vi "Parse POSCAR.vi"(8 "error in (no error)":errorcluster, 10 "POSCAR Type":string(combo)="Unknown", 11 "POSCAR File":path) -> (0 "error out":errorcluster, 1 "Summary Values":string[](array[string])=["# Atoms", "Cell Volume (A^3)", "|C|"], 2 "Summary Headers":string[](array[string])=["# Atoms", "Cell Volume (A^3)", "|A| (Å)", "|B| (Å)", "|C| (Å)", "alpha (deg)", "beta (deg)", "gamma (deg)"], 3 "Structure":T1)   [LabVIEW 2010]
uses:
  <vilib>/Analysis/baseanly.llb/Real Dot Product.vi
  <vilib>/Analysis/_algsub.llb/Real Vector Norm.vi
  <vilib>/Analysis/NI_AALPro.lvlib
  <vilib>/Analysis/NI_AALBase.lvlib
panel:
  out "element":string
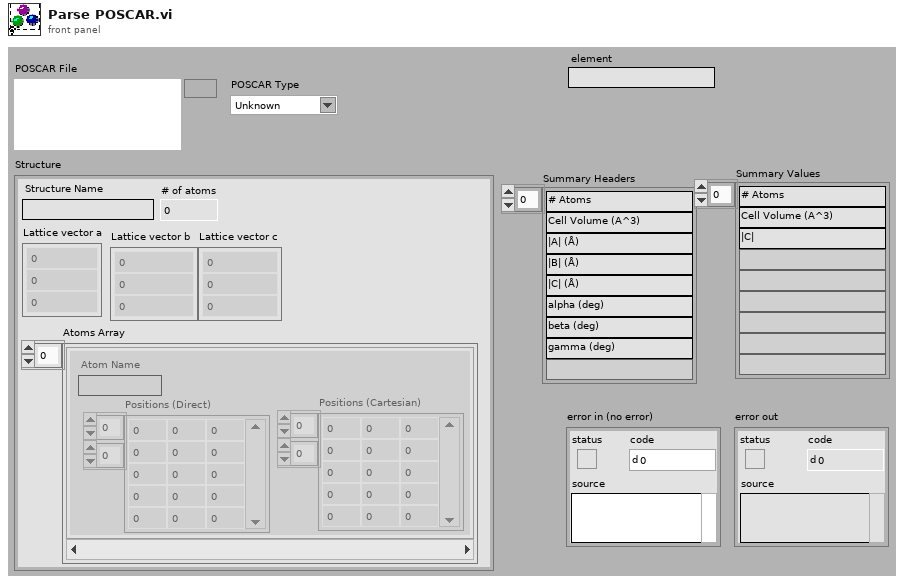
[diagram p1: front panel]
types:
  T1 = cluster{"Structure Name":string, "Lattice vector a":dbl[], "Lattice vector b":dbl[], "Lattice vector c":dbl[], "Atoms Array":cluster{"Atom Name":string, "Positions (Direct)":dbl[][], "Positions (Cartesian)":dbl[][]}[], "# of atoms":i32}
  T2 = cluster{"trimmed string":string, dbl[], dbl[], dbl[], cluster{string, dbl[][], dbl[][]}[], "token string":dbl}
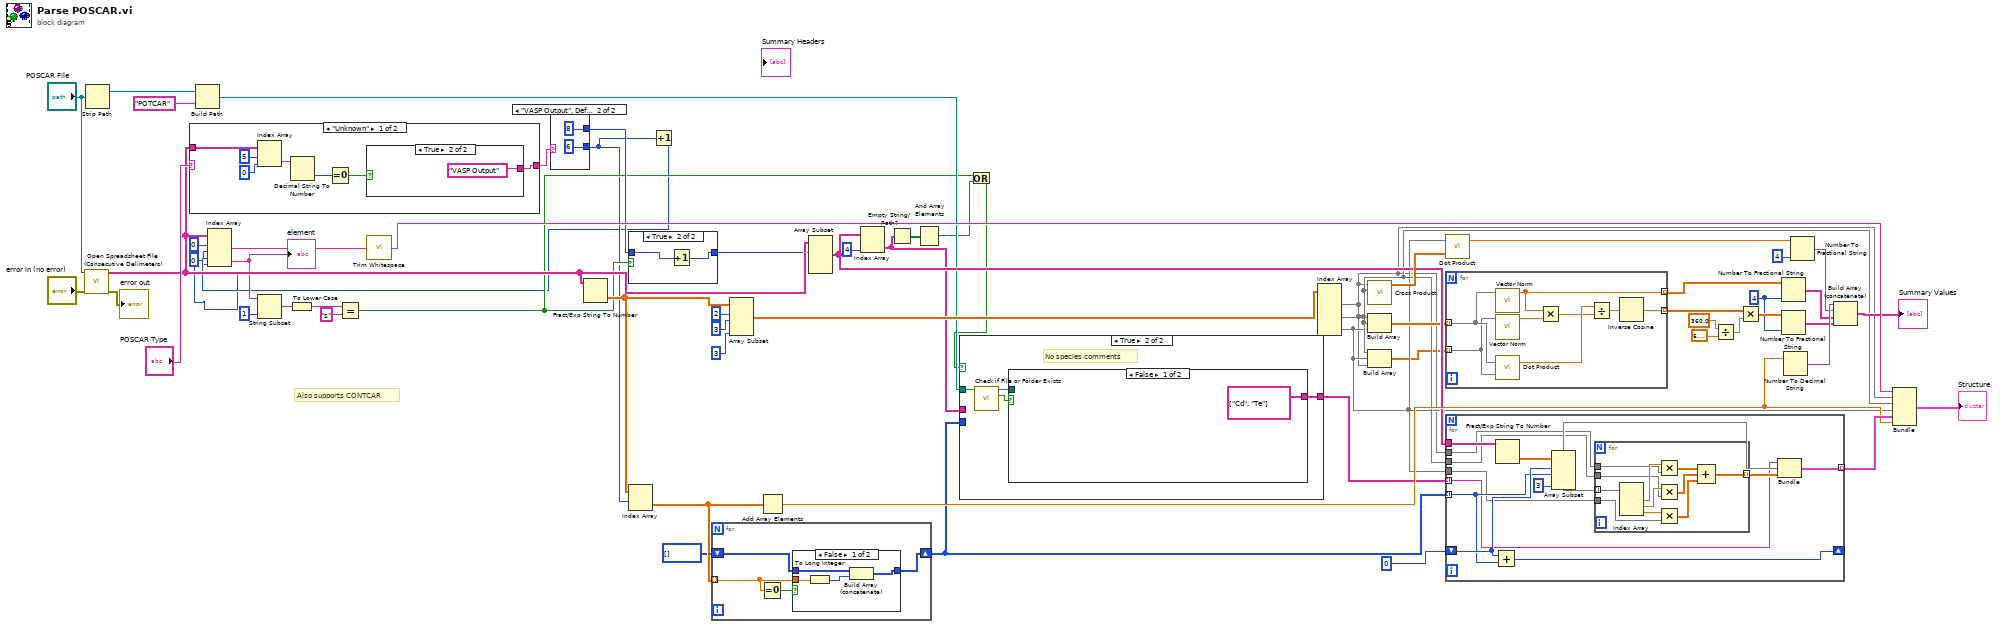
[diagram p0: block diagram]
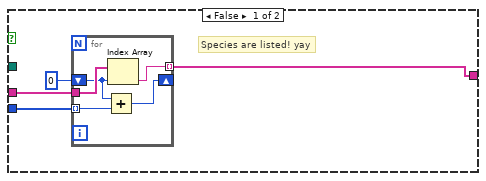
[diagram p3: hidden frame]
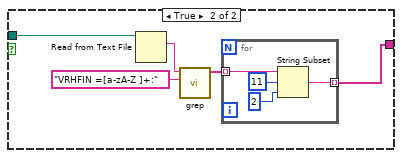
[diagram p4: hidden frame]
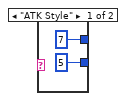
[diagram p6: hidden frame]
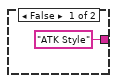
[diagram p7: hidden frame]
diagram:
  w20 = i16 4 ("precision (6)")
  w1 = 0 ("disabled index (col)")
  # "Also supports CONTCAR"
  n1 = call "Open Spreadsheet File (Consecutive Delimeters).vi"("error in (no error)"="error in (no error)", "File"="POSCAR File") -> ("error out"=→"error out":errorcluster, "Array"=w14:string[][])  [unwired: 8 in]
  n2 = Strip Path(path="POSCAR File") -> (stripped path=w40:path)  [unwired: 1 out]
  n3 = case shown="\"Unknown\"" "POSCAR Type" {
    selector: "POSCAR Type" -> [_ w72]
    tunnel: w14 -> [w69 _]
    tunnel: [w63 w72] -> w60
    frame "Unknown" {
      n4 = Index Array(array=w69, index (row)=5, index (col)=0 ("disabled index (col)")) -> (element=w66:string)
      n5 = Decimal String To Number(string=w66) -> (number=w65:i32)  [unwired: 2 in, 1 out]
      n6 = Equal To 0?(x=w65) -> (x = 0?=w64:bool)
      n7 = case shown="True" w64 {
        tunnel: ["ATK Style" "VASP Output"] -> w63
        frame False {
        }
        frame True {
        }
      }
    }
    frame Default {
    }
  }
  n8 = Build Path(base path=w40, name or relative path="POTCAR") -> (appended path=w36:path)
  n9 = case shown="\"VASP Output\", Default" w60 {
    tunnel: [5 ("index (row)") 6 ("index (row)")] -> w3
    tunnel: [7 ("index") 8 ("index")] -> w9
    frame "ATK Style" {
    }
    frame "VASP Output", Default {
    }
  }
  n10 = Fract/Exp String To Number(string=w14) -> (number=w15:dbl[][])  [unwired: 3 in, 1 out]
  n11 = Index Array(array=w15, index (row)=w3) -> (element=w59:dbl[])  [unwired: 1 in]
  n12 = Increment(x=w3) -> (x+1=w2:i32)
  n13 = Index Array(array=w14, index (row) #1=0 ("index (row)"), index (col) #1=w1, index (row) #2=w2, index (col) #2=w1) -> (element #1=w42:string, element #2=w7:string)
  "element" <- w7
  n14 = String Subset(string=w7, length (rest)=1 ("length (rest)")) -> (substring=w13:string)  [unwired: 1 in]
  n15 = To Lower Case(string=w13) -> (all lower case string=w11:string)
  n16 = Equal?(x=w11, y="s") -> (x = y?=w4:bool)
  n17 = call <vilib>:"Trim Whitespace.vi"("string"=w42) -> ("trimmed string"=w50:string)  [unwired: 1 in]
  n18 = case shown="True" w4 {
    tunnel: w9 -> [w77 w79]
    tunnel: [w77 w78] -> w8
    frame False {
    }
    frame True {
      n19 = Increment(x=w79) -> (x+1=w78:i32)
    }
  }
  n20 = for {
    tunnel: w59 -> [w82] mode=indexing
    shift-right: [w81] -> w35
    shift-left: i32[] [] -> [w80]
    n21 = Equal To 0?(x=w82) -> (x = 0?=w83:bool)
    n22 = case shown="False" w83 {
      tunnel: w82 -> [w87 _]
      tunnel: [w85 w88] -> w81
      tunnel: w80 -> [w84 w88]
      frame False {
        n23 = To Long Integer(number=w87) -> (32bit integer=w86:i32)
        n24 = Build Array (concatenate)(w84, w86) -> (w85:i32[])
      }
      frame True {
      }
    }
  }
  n25 = Array Subset(array=w15, index (row)=2, length (row)=3 ("length"), length (col)=3 ("length")) -> (w54:dbl[][])  [unwired: 1 in]
  n26 = Add Array Elements(numeric array=w59) -> (sum=w44:dbl)
  n27 = Array Subset(array=w14, index (row)=w8) -> (w38:string[][])  [unwired: 3 in]
  n28 = Index Array(array=w38, index (col)=4 ("disabled index (col)")) -> (element=w33:string[])  [unwired: 1 in]
  n29 = Empty String/Path?(string/path=w33) -> (empty?=w32:bool[])
  n30 = And Array Elements(Boolean array=w32) -> (logical AND=w6:bool)
  n31 = Or(x=w4, y=w6) -> (x .or. y?=w5:bool)
  n32 = case shown="True" w5 {
    tunnel: w36 -> [_ w101]
    tunnel: w33 -> [w92 _]
    tunnel: [w90 w98] -> w34
    tunnel: w35 -> [w91 _]
    frame False {
      # "Species are listed! yay"
      n33 = for {
        tunnel: w92 -> [w97]
        tunnel: w91 -> [w95] mode=indexing
        tunnel: [w96] -> w90 mode=indexing
        shift-right: [w94] -> _
        shift-left: 0 -> [w93]
        n34 = Add(x=w93, y=w95) -> (x+y=w94:i32)
        n35 = Index Array(array=w97, index=w93) -> (element=w96:string)
      }
    }
    frame True {
      # "No species comments"
      n36 = call <vilib>:"Check if File or Folder Exists.vi"("path"=w101) -> ("file or folder exists?"=w100:bool, "dup path"=w99:path)  [unwired: 8 in, 1 out]
      n37 = case shown="False" w100 {
        tunnel: w99 -> [_ w106]
        tunnel: [string[] ["Cd", "Te"] w103] -> w98
        frame False {
        }
        frame True {
          n38 = Read from Text File(file (use dialog)=w106) -> (text=w105:string)  [unwired: 3 in, 3 out]
          n39 = call "grep.vi"("Keyword (Regular Expression)"="VRHFIN =[a-zA-Z ]+:", "File String"=w105) -> ("Result"=w104:string[])  [unwired: 9 in]
          n40 = for {
            tunnel: w104 -> [w111] mode=indexing
            tunnel: [w108] -> w103 mode=indexing
            n41 = String Subset(string=w111, offset (0)=11, length (rest)=2 ("length (rest)")) -> (substring=w108:string)
          }
        }
      }
    }
  }
  n42 = Index Array(array=w54) -> (element #1=w28:dbl[], element #2=w30:dbl[], element #3=w29:dbl[])  [unwired: 6 in]
  n43 = call <vilib>:"Cross Product.vi"("B Vector"=w30, "A Vector"=w28) -> ("Cross Product"=w45:dbl[])  [unwired: 8 in, 1 out]
  n44 = Build Array(w28, w30, w29) -> (w31:dbl[][])
  n45 = Build Array(w30, w29, w28) -> (w27:dbl[][])
  n46 = call-poly <vilib>:"Dot Product.vi"("Y Vector"=w45, "X Vector"=w29) -> ("X * Y"=w48:dbl)  [unwired: 1 out]
  n47 = for {
    tunnel: w31 -> [w118] mode=indexing
    tunnel: w27 -> [w117] mode=indexing
    tunnel: [w115] -> w26 mode=indexing
    tunnel: [w112] -> w23 mode=indexing
    n48 = call-poly <vilib>:"Vector Norm.vi"("Input Vector"=w118) -> ("norm"=w115:dbl)  [unwired: 9 in, 1 out]
    n49 = call-poly <vilib>:"Vector Norm.vi"("Input Vector"=w117) -> ("norm"=w116:dbl)  [unwired: 9 in, 1 out]
    n50 = call-poly <vilib>:"Dot Product.vi"("Y Vector"=w117, "X Vector"=w118) -> ("X * Y"=w119:dbl)  [unwired: 1 out]
    n51 = Multiply(x=w115, y=w116) -> (x*y=w114:dbl)
    n52 = Divide(x=w119, y=w114) -> (x/y=w113:dbl)
    n53 = Inverse Cosine(1:w113) -> (0:w112:dbl)
  }
  n54 = for {
    tunnel: w38 -> [w127]
    tunnel: w35 -> [w129] mode=indexing
    shift-right: [w128] -> _
    shift-left: 0 ("length") -> [w130]
    tunnel: [w131] -> w52 mode=indexing
    tunnel: w28 -> [w125]
    tunnel: w30 -> [w124]
    tunnel: w29 -> [w123]
    tunnel: w34 -> [w121] mode=indexing
    n55 = Add(x=w130, y=w129) -> (x+y=w128:i32)
    n56 = Fract/Exp String To Number(string=w127) -> (number=w120:dbl[][])  [unwired: 3 in, 1 out]
    n57 = Array Subset(array=w120, index (row)=w130, length (row)=w129, length (col)=3 ("length")) -> (w126:dbl[][])  [unwired: 1 in]
    n58 = for {
      tunnel: w126 -> [w143] mode=indexing
      tunnel: w125 -> [w141]
      tunnel: w124 -> [w139]
      tunnel: w123 -> [w137]
      tunnel: [w133] -> w122 mode=indexing
      n59 = Index Array(array=w143) -> (element #1=w142:dbl, element #2=w140:dbl, element #3=w138:dbl)  [unwired: 3 in]
      n60 = Multiply(x=w142, y=w141) -> (x*y=w136:dbl[])
      n61 = Multiply(x=w140, y=w139) -> (x*y=w135:dbl[])
      n62 = Multiply(x=w138, y=w137) -> (x*y=w134:dbl[])
      n63 = Compound Arithmetic op=ADD(w136, w135, w134) -> (w133:dbl[])
    }
    n64 = Bundle(w121, w126, w122) -> (w131:cluster{string, dbl[][], dbl[][]})  [unwired: 1 in]
  }
  n65 = Divide(x=360.0, y=6.283185307179586) -> (x/y=w22:dbl)
  n66 = Multiply(x=w23, y=w22) -> (x*y=w21:dbl[])
  n67 = Number To Fractional String(number=w26, precision (6)=w20) -> (F-format string=w19:string[])  [unwired: 2 in]
  n68 = Number To Fractional String(number=w21, precision (6)=w20) -> (F-format string=w18:string[])  [unwired: 2 in]
  n69 = Number To Decimal String(number=w44) -> (decimal integer string=w49:string)  [unwired: 1 in]
  n70 = Number To Fractional String(number=w48, precision (6)=i16 4) -> (F-format string=w46:string)  [unwired: 2 in]
  n71 = Build Array (concatenate)(w49, w46, w19, w18) -> (→"Summary Values":string[])
  n72 = Bundle("trimmed string"=w50, w28, w30, w29, w52, "token string"=w44) -> (→"Structure":T2)  [unwired: 1 in]
